vi "GT Get Var Bool Condition.vi"(8 "error in (no error)":errorcluster caption="错误输入（无错误）", 9 "pWatchCondition":T1, 10 "varIndex":i16, 11 "cardNum":i16) -> (0 "error out":errorcluster caption="错误输出", 1 "pWatchCondition out":T1, 3 "function return":i16)   [LabVIEW 2020, in "gts1.lvlib"]
doc: "GT_API GT_GetVarBoolCondition(short cardNum,short varIndex,TWatchCondition *pWatchCondition);"
uses:
  gts1.lvlib
  dll/32bit/multi_card/gts.dll
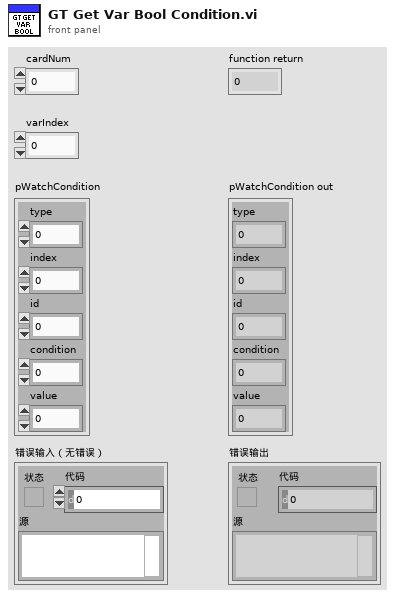
[diagram p1: front panel]
types:
  T1 = cluster{"type":u16, "index":u16, "id":u16, "condition":u16, "value":dbl}
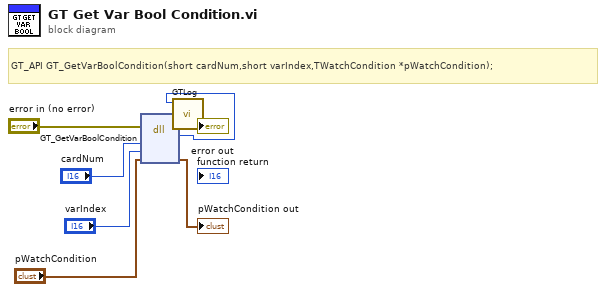
[diagram p0: block diagram]
diagram:
  # "GT_API GT_GetVarBoolCondition(short cardNum,short varIndex,TWatchCondition *pWatchCondition);"
  n1 = dll-call lib="C:/1228/dll/32bit/multi_card/gts.dll" fn="GT_GetVarBoolCondition"(error in="error in (no error)", "cardNum"="cardNum", "varIndex"="varIndex", "pWatchCondition"="pWatchCondition") -> (error out=w3:errorcluster, w1:i16, "pWatchCondition"=→"pWatchCondition out":T1)  [unwired: 4 in, 1 out]
  n2 = call "GTLog.vi"("error in (no error)"=w3, "Numeric"=w1) -> ("error out"=→"error out":errorcluster)  [unwired: 9 in]
